vi "Charging State Log.vi"(6 "Timestamp":string[](array[string])=["00:00", "00:01", "00:02"], 7 "Charging State":string[](array[string])=["CHARGE_CC_SLOW-3", "CHARGE_CC_SLOW-3", "CHARGE_CC_SLOW-3"], 8 "error in":errorcluster, 9 "Rcvd Level":dbl[](array[numeric])=[100.0, 101.0, 99.0], 10 "Temp Level":dbl[](array[numeric])=[3.0, 4.0, 4.0], 11 "IPG Temp":dbl[](array[numeric])=[35.0, 35.1, 35.2] format="%.2f") -> (0 "error out":errorcluster)   [LabVIEW 2010]
uses:
  Drivers/Telemetry/MICS_ID Global.vi
panel:
  in  "results file":path=path "C:/ATS Reports/Charging Test Results_"
  in  "Temperature Data Log":string[][](table)=[["", "", "", "", ""], ["", "", "", "", ""], ["", "", "", "", ""]] caption="Table 1"
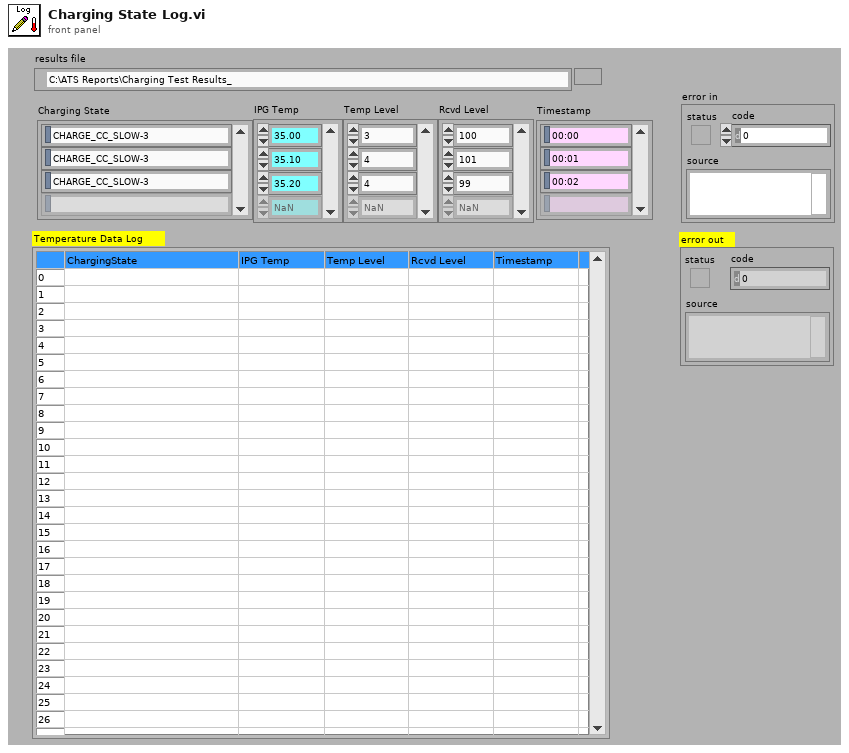
[diagram p1: front panel]
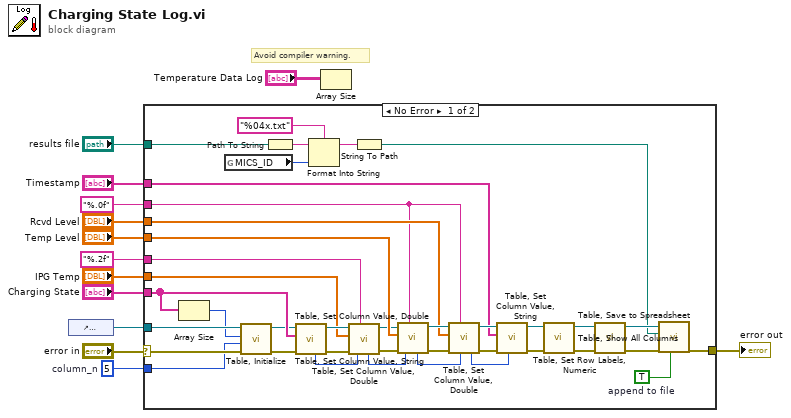
[diagram p0: block diagram]
diagram:
  w1 = 5  # column_n
  # "Avoid compiler warning."
  n1 = control-ref of="Temperature Data Log"() -> (w13:refnum<vi>)
  n2 = case shown="No Error" "error in" {
    selector: "error in" -> [w29 w53]
    tunnel: w13 -> [w27 _]
    tunnel: "Charging State" -> [w50 _]
    tunnel: "Rcvd Level" -> [w46 _]
    tunnel: "Temp Level" -> [w41 _]
    tunnel: "%.0f" ("format (%f)") -> [w38 _]
    tunnel: "IPG Temp" -> [w37 _]
    tunnel: [w22 w53] -> w6
    tunnel: "results file" -> [w19 _]
    tunnel: "%.2f" ("format (%f)") -> [w36 _]
    tunnel: "Timestamp" -> [w30 _]
    tunnel: w1 -> [w25 _]
    frame No Error {
      w20 = TRUE  # append to file
      n3 = Array Size(array=w50) -> (size(s)=w26:i32)
      n4 = global read "MICS_ID Global.vi" "MICS_ID"() -> (w16:u32)
      n5 = call "Table, Initialize.vi"("error in"=w29, "column_n (0)"=w25, "row_n (0)"=w26, "Tbl Refnum"=w27) -> ("error out"=w28:errorcluster, "Tbl Refnum dup"=w24:refnum<vi>)  [unwired: 6 in]
      n6 = Path To String(path=w19) -> (string=w17:string)
      n7 = call "Table, Set Column Value, String.vi"("error in"=w28, "Value"=w50, "Tbl Refnum"=w24) -> ("error out"=w44:errorcluster, "Tbl Refnum out"=w40:refnum<vi>, "column+1"=w43:i32)  [unwired: 6 in]
      n8 = Format Into String(format string="%04x.txt", initial string=w17, w16) -> (resulting string=w14:string)  [unwired: 1 in, 1 out]
      n9 = call "Table, Set Column Value, Double.vi"("column (0)"=w43, "format (%f)"=w36, "error in"=w44, "Value"=w37, "Tbl Refnum"=w40) -> ("error out"=w45:errorcluster, "Tbl Refnum out"=w39:refnum<vi>, "column+1"=w42:i32)  [unwired: 4 in]
      n10 = String To Path(string=w14) -> (path=w18:path)
      n11 = call "Table, Set Column Value, Double.vi"("column (0)"=w42, "format (%f)"=w38, "error in"=w45, "Value"=w41, "Tbl Refnum"=w39) -> ("error out"=w49:errorcluster, "Tbl Refnum out"=w47:refnum<vi>, "column+1"=w48:i32)  [unwired: 4 in]
      n12 = call "Table, Set Column Value, Double.vi"("column (0)"=w48, "format (%f)"=w38, "error in"=w49, "Value"=w46, "Tbl Refnum"=w47) -> ("error out"=w35:errorcluster, "Tbl Refnum out"=w33:refnum<vi>, "column+1"=w31:i32)  [unwired: 4 in]
      n13 = call "Table, Set Column Value, String.vi"("column (0)"=w31, "error in"=w35, "Value"=w30, "Tbl Refnum"=w33) -> ("error out"=w34:errorcluster, "Tbl Refnum out"=w32:refnum<vi>)  [unwired: 5 in, 1 out]
      n14 = call "Table, Show All Columns.vi"("error in"=w34, "Tbl Refnum"=w32) -> ("error out"=w52:errorcluster, "Tbl Refnum out"=w51:refnum<vi>)  [unwired: 8 in]
      n15 = call "Table, Set Row Labels, Numeric.vi"("error in"=w52, "Tbl Refnum"=w51) -> ("error out"=w23:errorcluster, "Tbl Refnum out"=w21:refnum<vi>)  [unwired: 8 in]
      n16 = call "Table, Save to Spreadsheet.vi"("append to file (F)"=w20, "error in"=w23, "spreadsheet file"=w18, "Tbl Refnum"=w21) -> ("error out"=w22:errorcluster)  [unwired: 4 in, 1 out]
    }
    frame Error {
    }
  }
  "error out" <- w6
  n17 = Array Size(array="Temperature Data Log") -> ()  [unwired: 1 out]
